vi "PMTread.vi"(11 "PMT Settings":cluster{"Bin Length":dbl, "Show Mean":bool}) -> ()   [LabVIEW 2017]
uses:
  <vilib>/Utility/error.llb/Error Cluster From Error Code.vi
  <vilib>/rvi/errors/niLvFpgaAdjustHostInterfaceError.vi
  <vilib>/rvi/interface/nirviReadWriteControl/nirviReadWriteControl.xnode
  NiFpgaLv.dll
  <vilib>/rvi/interface/Simulation/niFpgaSimulationCallBeginRW.vi
panel:
  in  "error in":errorcluster
  out "PMT saturation":bool
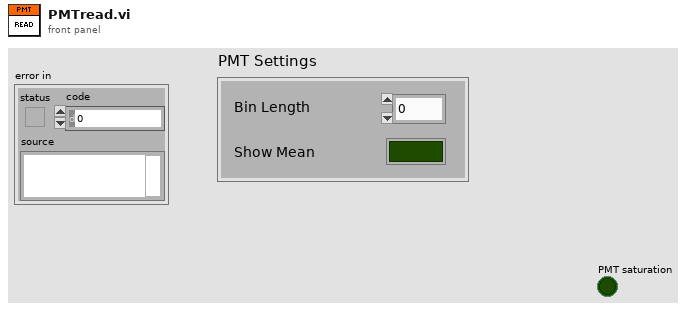
[diagram p1: front panel]
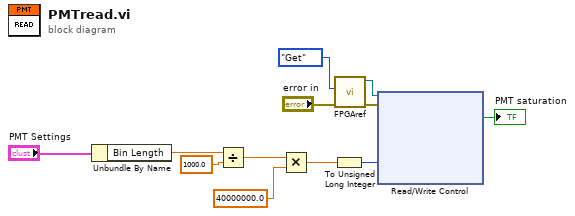
[diagram p0: block diagram]
diagram:
  n1 = Unbundle By Name("PMT Settings") -> ("Bin Length"=w4:dbl)
  n2 = Divide(x=w4, y=1000.0) -> (x/y=w6:dbl)
  n3 = Multiply(x=w6, y=40000000.0) -> (x*y=w3:dbl)
  n4 = To Unsigned Long Integer(number=w3) -> (unsigned 32bit integer=w2:u32)
  n5 = call "FPGAref.vi"("error in"="error in", "Enum"=enum16{"Set", "Get"}."Get") -> ("error out"=w8:errorcluster, "FPGA VI Reference Out 2"=w9:refnum<k20>)  [unwired: 4 in]
  n6 = xnode "Read/Write Control"("FPGA VI Reference In"=w9, "error in"=w8, "ticks per bin"=w2) -> ("PMT saturation"=→"PMT saturation":bool)  [unwired: 5 out]
